vi "LLen.vi"(0 "reference in":refnum<class "Redis.lvclass">, 1 "Key":string, 11 "Error In":errorcluster) -> (4 "reference out":refnum<class "Redis.lvclass">, 8 "Length":i64, 15 "Error Out":errorcluster)   [LabVIEW 2020, in "Redis.lvclass"]
doc: "<b>LLEN</b>\n\nReturns the length of the list stored at key. If key does not exist, it is interpreted as an empty list and 0 is returned. An error is returned when the value stored at key is not a list."
uses:
  Redis.lvclass
  Redis.lvclass/Redis.ctl
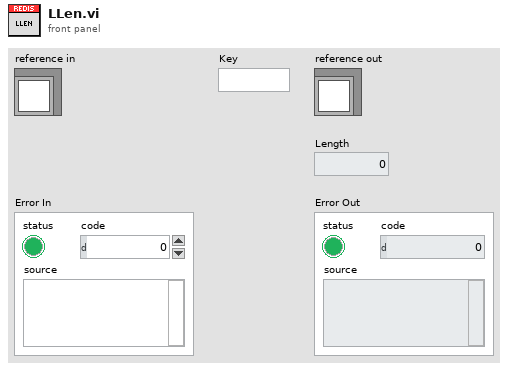
[diagram p1: front panel]
types:
  T1 = typedef "Redis.lvclass/RedisDataType.ctl" = cluster{"Reply Type":T2, "Integer":i64, "String":string, "Multibulk":variant[], "StringData":string[]}
  T2 = typedef "Redis.lvclass/ReplyDataTypeEnum.ctl" = enum16{"None", "Error", "Status", "Nil", "Integer", "String", "Multibulk"}
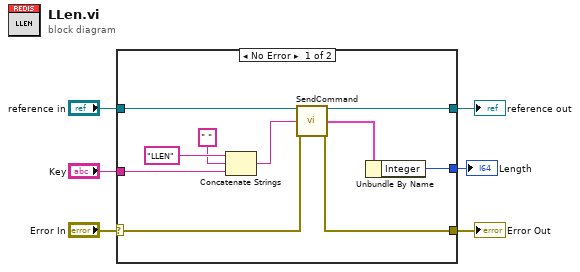
[diagram p0: block diagram]
diagram:
  n1 = case shown="No Error" "Error In" {
    selector: "Error In" -> [w14 w18]
    tunnel: [w13 w18] -> w5
    tunnel: [w16 w17] -> w3
    tunnel: "reference in" -> [w15 w17]
    tunnel: "Key" -> [w11 _]
    tunnel: [w7 _] -> w1
    frame No Error {
      n2 = Concatenate Strings("LLEN", " ", w11) -> (w10:string)
      n3 = call "SendCommand.vi"("reference in"=w15, "Command"=w10, "Error In"=w14) -> ("reference out"=w16:refnum<class "Redis.lvclass">, "Data"=w8:T1, "Error Out"=w13:errorcluster)  [unwired: 10 in]
      n4 = Unbundle By Name(w8) -> ("Integer"=w7:i64)
    }
    frame Error {
    }
  }
  "Error Out" <- w5
  "reference out" <- w3
  "Length" <- w1
